vi "DataPacker_QueueInspector.vi"() -> ()   [LabVIEW 2018, in "feGEM DataPacker.lvlib"]
uses:
  DataStructures/GEM_BANK_CLUSTER_typedef.ctl
  DataStructures/GEM_DATA_cluster_typedef.ctl
  feGEM DataPacker.lvlib
panel:
  out "Array Size":dbl[](array[numeric])
  out "Bytes in data payload":i32[](array[numeric])
  out "Timestamp":timestamp[](array[timestamp]) format="%<%H:%M:%S%7u>T"
  out "Array Data (Array being logged)":string[](array[string])
  out "Data type":string[](array[string])
  out "Write to MIDAS history database every N seconds":u16[](array[numeric])
  out "Bitwise history settings":u16[](array[numeric])
  out "Equipment description (31 char limit)":string[](array[string])
  out "Queue Position":i32[](array[numeric])
  out "Variable (15 char limit)":string[](array[string])
  out "Category (15 char limit)":string[](array[string])
  in  "Stop full data inspector (heavy)":bool
  out "max queue size":i32
  out "# elements in queue":i32
  in  "Stop Queue Length Reader (lightweight)":bool
  out "Seconds since last communication with MIDAS (should remain below 2 seconds)":dbl
  out "MIDAS Connection OK":bool
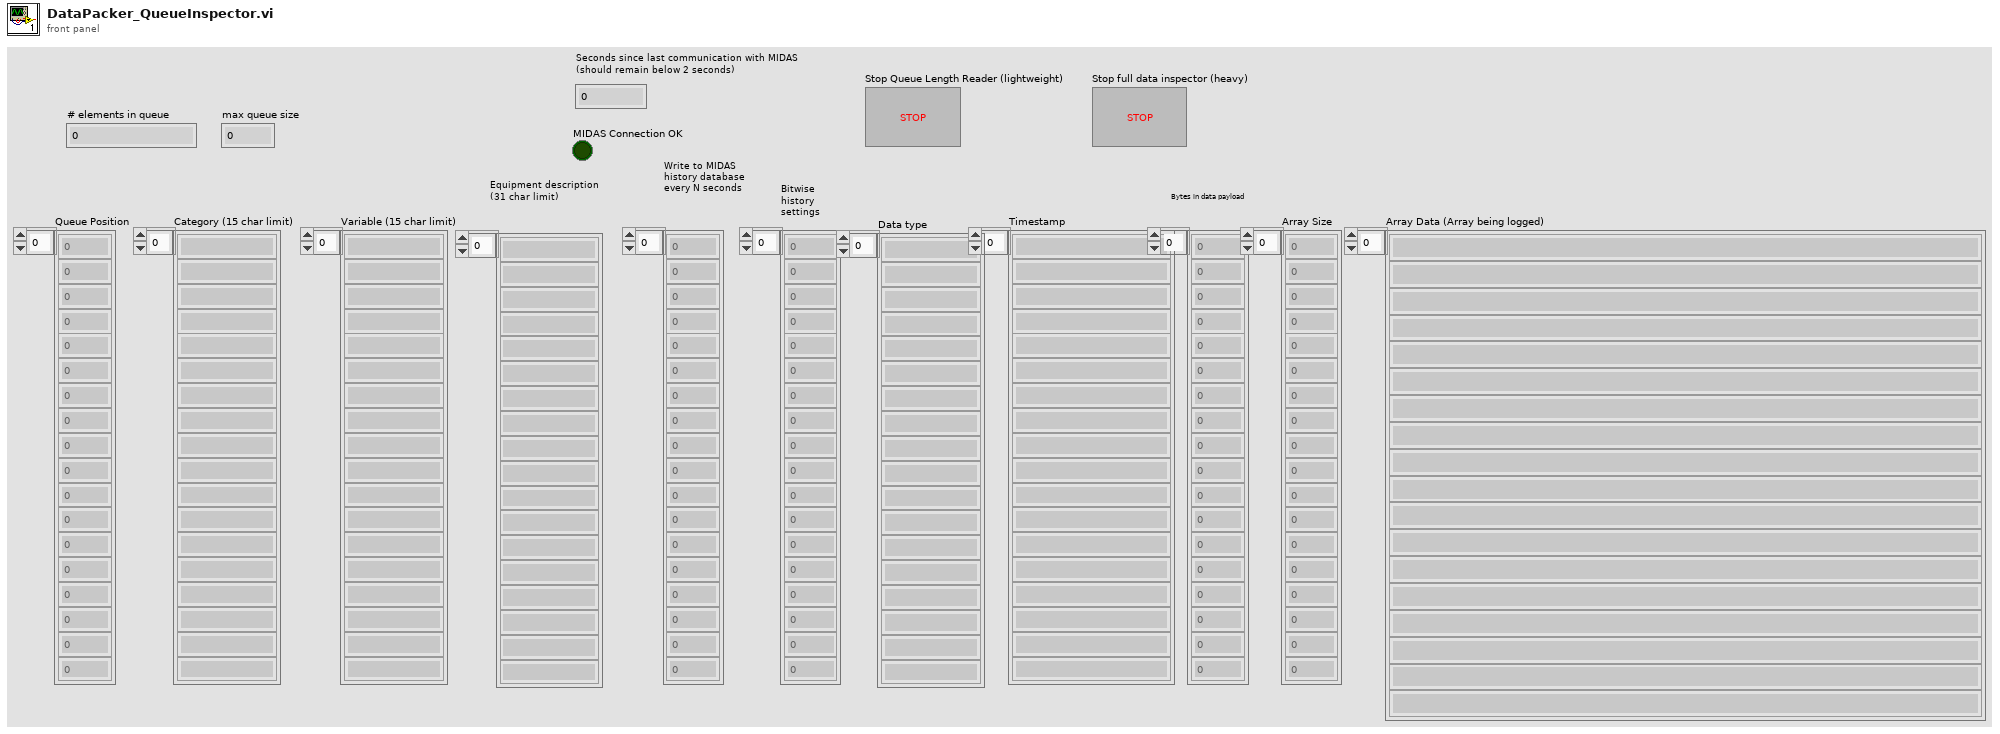
[diagram p1: front panel]
types:
  T1 = typedef "feGEM DataPacker.lvlib/GEM_BANK_CLUSTER_typedef.ctl" = cluster{"Category":string, "Variable Name":string, "Equipment description":string, "History Settings":u16, "Period to update history plots":u16, "GEM_DATA Cluster":T2}
  T2 = typedef "feGEM DataPacker.lvlib/GEM_DATA_cluster_typedef.ctl" = cluster{"DataType":string, "Formatted Data":u8[], "data byte order (Little Endian prefered)":enum16{"big-endian, network order", "native, host order", "little-endian"}}
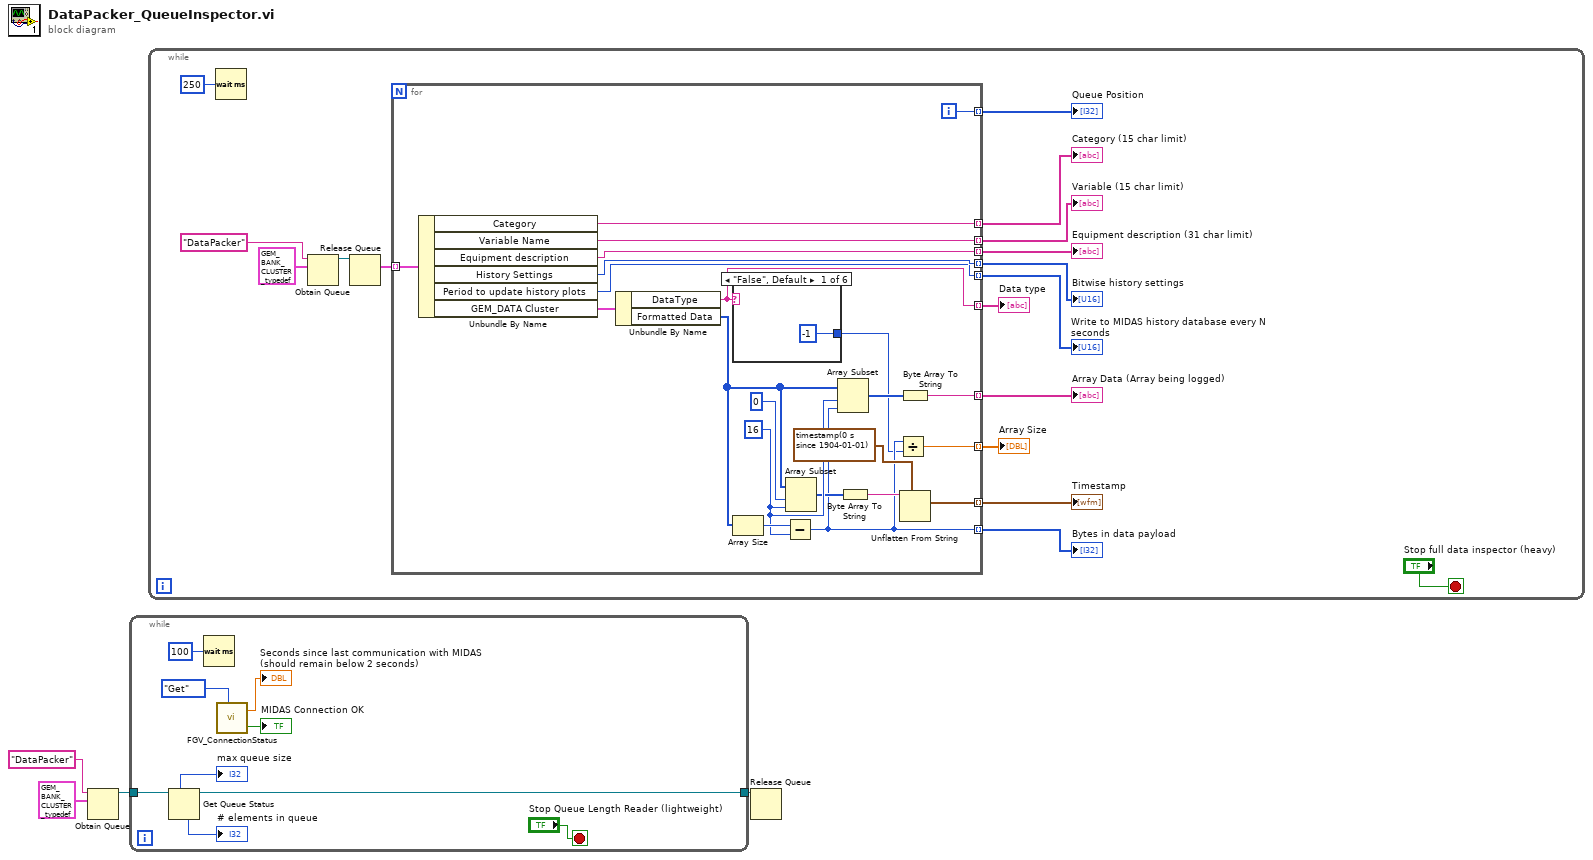
[diagram p0: block diagram]
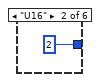
[diagram p2: hidden frame]
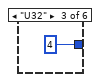
[diagram p3: hidden frame]
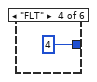
[diagram p4: hidden frame]
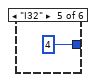
[diagram p5: hidden frame]
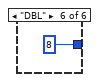
[diagram p6: hidden frame]
diagram:
  n1 = Obtain Queue(name (unnamed)="DataPacker", element data type=T1 {"Category"="", "Variable Name"="", "Equipment description"="", "History Settings"=0, "Period to update history plots"=0, "GEM_DATA Cluster"={"DataType"="", "Formatted Data"=[], "data byte order (Little Endian prefered)"=enum."big-endian, network order"}} ("output cluster")) -> (queue out=w2:refnum<queue>)  [unwired: 3 in, 2 out]
  n2 = while {
    tunnel: w2 -> [w8]
    tunnel: [w5] -> w1
    stop <- "Stop Queue Length Reader (lightweight)" stop-if-true
    n3 = Get Queue Status(queue=w8) -> (queue out=w5:refnum<queue>, max queue size=→"max queue size":i32, # elements in queue=→"# elements in queue":i32)  [unwired: 2 in, 5 out]
    n4 = Wait (ms)(milliseconds to wait=u32 100) -> ()  [unwired: 1 out]
    n5 = call "FGV_ConnectionStatus.vi"("Enum"=enum16{"Get", "Set"}."Get") -> ("Seconds since last communication with MIDAS"=→"Seconds since last communication with MIDAS (should remain below 2 seconds)":dbl, "MIDAS Connection OK"=→"MIDAS Connection OK":bool)  [unwired: 4 in]
  }
  n6 = while {
    stop <- "Stop full data inspector (heavy)" stop-if-true
    n7 = Wait (ms)(milliseconds to wait=u32 250) -> ()  [unwired: 1 out]
    n8 = Obtain Queue(name (unnamed)="DataPacker", element data type=T1 {"Category"="", "Variable Name"="", "Equipment description"="", "History Settings"=0, "Period to update history plots"=0, "GEM_DATA Cluster"={"DataType"="", "Formatted Data"=[], "data byte order (Little Endian prefered)"=enum."big-endian, network order"}} ("output cluster")) -> (queue out=w28:refnum<queue>)  [unwired: 3 in, 2 out]
    n9 = Release Queue(queue=w28) -> (remaining elements=w26:T1[])  [unwired: 2 in, 2 out]
    n10 = for {
      tunnel: w26 -> [w52] mode=indexing
      tunnel: [w51] -> w24 mode=indexing
      tunnel: [w50] -> w23 mode=indexing
      tunnel: [w49] -> w22 mode=indexing
      tunnel: [w48] -> w21 mode=indexing
      tunnel: [w47] -> w20 mode=indexing
      tunnel: [w46] -> w19 mode=indexing
      tunnel: [w34] -> w18 mode=indexing
      tunnel: [w42] -> w17 mode=indexing
      tunnel: [w35] -> w16 mode=indexing
      tunnel: [w33] -> w15 mode=indexing
      tunnel: [w31] -> w14 mode=indexing
      i -> [w49]
      w40 = 16 ("y")
      n11 = Unbundle By Name(w52) -> ("Category"=w51:string, "Variable Name"=w50:string, "Equipment description"=w48:string, "History Settings"=w47:u16, "Period to update history plots"=w46:u16, "GEM_DATA Cluster"=w45:T2)
      n12 = Unbundle By Name(w45) -> ("DataType"=w34:string, "Formatted Data"=w43:u8[])
      n13 = case shown="\"False\", Default" w34 {
        tunnel: [-1 ("y") 2 ("y") 4 ("y") 4 4 ("y") 8 ("y")] -> w32
        frame "False", Default {
        }
        frame "U16" {
        }
        frame "U32" {
        }
        frame "FLT" {
        }
        frame "I32" {
        }
        frame "DBL" {
        }
      }
      n14 = Array Size(array=w43) -> (size(s)=w44:i32)
      n15 = Subtract(x=w44, y=w40) -> (x-y=w33:i32)
      n16 = Array Subset(array=w43, index=0, length=w40) -> (w38:u8[])
      n17 = Array Subset(array=w43, index=w40, length=w33) -> (w39:u8[])
      n18 = Byte Array To String(unsigned byte array=w38) -> (string=w37:string)
      n19 = Divide(x=w33, y=w32) -> (x/y=w31:dbl)
      n20 = Byte Array To String(unsigned byte array=w39) -> (string=w42:string)
      n21 = Unflatten From String(type=timestamp(0 s since 1904-01-01), binary string=w37) -> (value=w35:timestamp)  [unwired: 3 in, 2 out]
    }
    "Category (15 char limit)" <- w24
    "Variable (15 char limit)" <- w23
    "Queue Position" <- w22
    "Equipment description (31 char limit)" <- w21
    "Bitwise history settings" <- w20
    "Write to MIDAS history database every N seconds" <- w19
    "Data type" <- w18
    "Array Data (Array being logged)" <- w17
    "Timestamp" <- w16
    "Bytes in data payload" <- w15
    "Array Size" <- w14
  }
  n22 = Release Queue(queue=w1) -> ()  [unwired: 2 in, 3 out]
